vi "Parse Request.vi"(8 "error in (no error)":errorcluster, 10 "{JSON} Request":string, 11 "JSON-RPC in":refnum<class "JSON-RPC.lvclass">) -> (0 "error out":errorcluster, 1 "Params":string[](array[string]), 2 "Methods":string[](array[string]), 3 "JSON-RPC out":refnum<class "JSON-RPC.lvclass">, 4 "IDs":string[](array[string]))   [LabVIEW 2019, in "JSON-RPC.lvclass"]
uses:
  JSON-RPC.lvclass
  JSON-RPC.lvclass/JSON-RPC.ctl
  private/Parse Request-JSONtext.vi/523bbeac-5bfa-4355-a479-ec0e355c2dae.vi
  private/Parse Request-JSONtext.vi/5dfc14ef-dff6-4e36-b5f1-09fb62becacc.vi
  private/Parse Request-JSONtext.vi/f339b867-7010-45a6-b71e-b2a9da4366e1.vi
  <vilib>/JDP Science/JSONtext/Find Item.vi
  <vilib>/JDP Science/JSONtext/String Subset.vi
  <vilib>/JDP Science/JSONtext/Get all Object Items.vi
  <vilib>/JDP Science/JSONtext/Parsing/Parse Full Path or Item Name.vi
  <vilib>/JDP Science/JSONtext/Next JSON Value.vi
  <vilib>/JDP Science/JSONtext/support/Error Cluster From Code.vi
  <vilib>/JDP Science/JSONtext/Offset/Find Item Locations by Path.vi
  <vilib>/JDP Science/JSONtext/JSON text to Variant.vi
  <vilib>/JDP Science/JSONtext/LVClass Serializer/JSONtext LVClass Serializer.lvclass
  <vilib>/JDP Science/JSONtext/JSONtext.lvlib
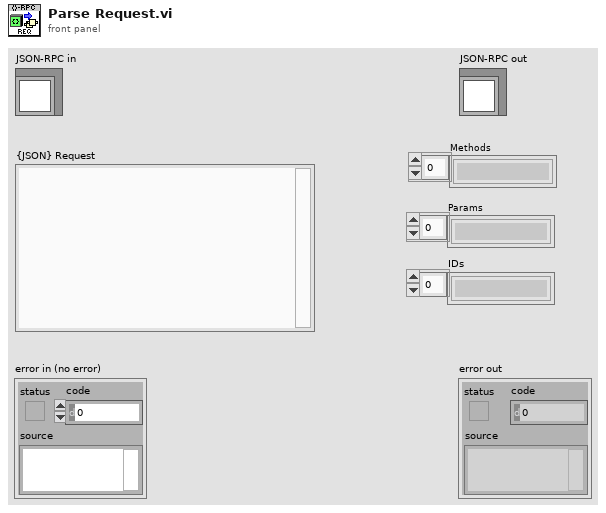
[diagram p1: front panel]
types:
  T1 = typedef "JSONtext.lvlib/JSON Value Type.ctl" = enum16{"Not a JSON Value", "JSON Object", "JSON Array", "String", "Number", "true", "false", "null"}
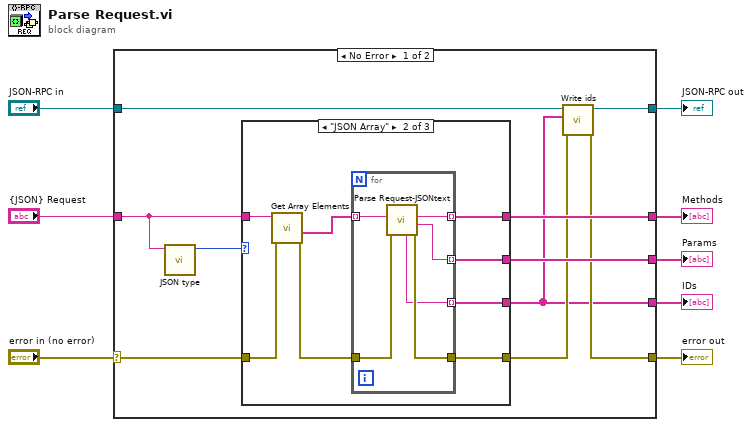
[diagram p0: block diagram]
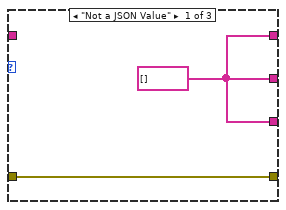
[diagram p2: hidden frame]
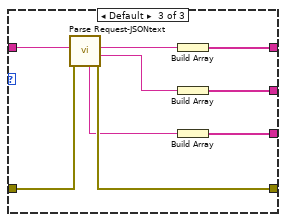
[diagram p3: hidden frame]
diagram:
  n1 = case shown="No Error" "error in (no error)" {
    selector: "error in (no error)" -> [w15 w45]
    tunnel: [w12 w45] -> w7
    tunnel: [w11 w44] -> w5
    tunnel: "JSON-RPC in" -> [w10 w44]
    tunnel: "{JSON} Request" -> [w14 _]
    tunnel: [w18 _] -> w2
    tunnel: [w17 _] -> w3
    tunnel: [w9 _] -> w1
    frame No Error {
      n2 = call <vilib>:"JSON type.vi"("JSON"=w14) -> ("JSON Value Type"=w16:T1)  [unwired: 9 in, 1 out]
      n3 = case shown="\"JSON Array\"" w16 {
        tunnel: w15 -> [w20 w24 w38]
        tunnel: [w20 w28 w37] -> w13
        tunnel: w14 -> [_ w25 w41]
        tunnel: [w19 w27 w43] -> w17
        tunnel: [w19 w26 w42] -> w18
        tunnel: [w19 w22 w35] -> w9
        frame "Not a JSON Value" {
          w19 = string[] []
        }
        frame "JSON Array" {
          n4 = call <vilib>:"Get Array Elements.vi"("error in (no error)"=w24, "JSON"=w25) -> ("error out"=w21:errorcluster, "<JSON>"=w23:string[])  [unwired: 7 in, 1 out]
          n5 = for {
            tunnel: w23 -> [w32] mode=indexing
            tunnel: [w31] -> w27 mode=indexing
            tunnel: [w29] -> w26 mode=indexing
            tunnel: [w30] -> w22 mode=indexing
            tunnel: w21 -> [w33]
            tunnel: [w34] -> w28
            n6 = call "Parse Request-JSONtext.vi"("error in (no error)"=w33, "{JSON} Request"=w32) -> ("error out"=w34:errorcluster, "params"=w29:string, "method"=w31:string, "id"=w30:string)  [unwired: 6 in]
          }
        }
        frame Default {
          n7 = call "Parse Request-JSONtext.vi"("error in (no error)"=w38, "{JSON} Request"=w41) -> ("error out"=w37:errorcluster, "params"=w39:string, "method"=w40:string, "id"=w36:string)  [unwired: 6 in]
          n8 = Build Array(w40) -> (w43:string[])
          n9 = Build Array(w39) -> (w42:string[])
          n10 = Build Array(w36) -> (w35:string[])
        }
      }
      n11 = call "Write ids.vi"("error in (no error)"=w13, "ids"=w9, "JSON-RPC in"=w10) -> ("error out"=w12:errorcluster, "JSON-RPC out"=w11:refnum<class "JSON-RPC.lvclass">)  [unwired: 7 in]
    }
    frame Error {
    }
  }
  "error out" <- w7
  "JSON-RPC out" <- w5
  "Methods" <- w3
  "Params" <- w2
  "IDs" <- w1
